vi "DestroyHttpSession.vi"(8 "error in":errorcluster, 11 "reQwestClient in":refnum<class "reQwestClient.lvclass">) -> (0 "error out":errorcluster)   [LabVIEW 2020, in "reQwestClient.lvclass"]
uses:
  reQwestClient.lvclass
  reQwestClient.lvclass/reQwestClient.ctl
  submodules/reqwest-rs-labview/lv_src/Client/Client.lvclass
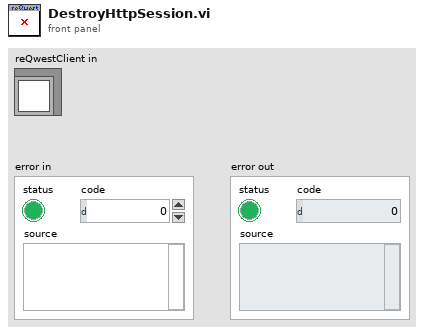
[diagram p1: front panel]
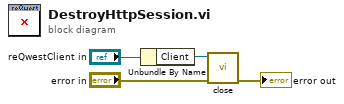
[diagram p0: block diagram]
diagram:
  n1 = Unbundle By Name("reQwestClient in") -> ("Client"=w3:refnum<class "Client.lvclass">)
  n2 = call "close.vi"("error in (no error)"="error in", "Client in"=w3) -> ("error out"=→"error out":errorcluster)  [unwired: 9 in]
